vi "PublishGamepad.vi"(6 "Buttons":bool[](array[boolean]), 8 "error in (no error)":errorcluster, 9 "Right Stick":cluster{"X":dbl, "Y":dbl}, 10 "Left Stick":cluster{"X":dbl, "Y":dbl}, 11 "JoystickDevRef":T1={"Device"=enum."USB 1"}) -> (0 "error out":errorcluster, 3 "JoystickDevRef":T1={"Device"=enum."USB 1"})   [LabVIEW 2014]
uses:
  <vilib>/Rock Robotics/WPI/Joystick/WPI_JoystickDevRef.ctl
  <vilib>/Rock Robotics/WPI/Joystick/WPI_JoystickDeviceEnum.ctl
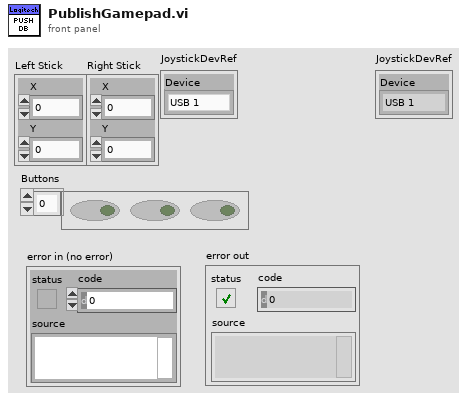
[diagram p1: front panel]
types:
  T1 = typedef "WPI_JoystickDevRef.ctl" = cluster{"Device":T2}
  T2 = typedef "WPI_JoystickDeviceEnum.ctl" = enum16{"USB 0", "USB 1", "USB 2", "USB 3", "USB 4", "USB 5"}
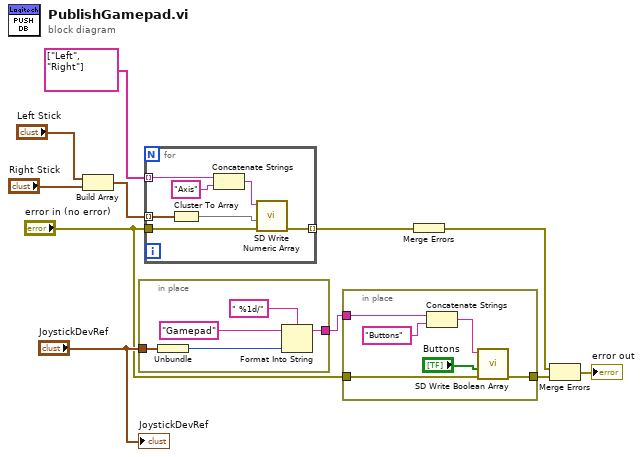
[diagram p0: block diagram]
diagram:
  n1 = Build Array("Left Stick", "Right Stick") -> (w10:cluster{"X":dbl, "Y":dbl}[])
  n2 = in-place {
    in-place-border: [w16] -> w6
    in-place-border: "JoystickDevRef" -> [w15]
    n3 = Unbundle(w15) -> ("Device"=w12:T2)
    n4 = Format Into String(format string=" %1d/", initial string="Gamepad", w12) -> (resulting string=w16:string)  [unwired: 1 in, 1 out]
  }
  n5 = for {
    tunnel: w10 -> [w20] mode=indexing
    tunnel: [w19] -> w9 mode=indexing
    tunnel: "error in (no error)" -> [w18]
    tunnel: string[] ["Left", "Right"] -> [w17] mode=indexing
    n6 = Cluster To Array(cluster=w20) -> (array=w22:dbl[])
    n7 = Concatenate Strings(w17, "Axis" ("string")) -> (w21:string)
    n8 = call <vilib>:"SD Write Numeric Array.vi"("error in"=w18, "Numeric Array"=w22, "Name"=w21) -> ("error out"=w19:errorcluster)  [unwired: 7 in, 1 out]
  }
  n9 = in-place {
    in-place-border: [w29] -> w11
    in-place-border: w6 -> [w28]
    in-place-border: "error in (no error)" -> [w27]
    n10 = Concatenate Strings(w28, "Buttons" ("string")) -> (w24:string)
    n11 = call <vilib>:"SD Write Boolean Array.vi"("error in"=w27, "Boolean Array"="Buttons", "Name"=w24) -> ("error out"=w29:errorcluster)  [unwired: 7 in, 1 out]
  }
  n12 = Merge Errors(w9) -> (w8:errorcluster)
  n13 = Merge Errors(w8, w11) -> (→"error out":errorcluster)
  "JoystickDevRef" <- "JoystickDevRef"
